vi "Promedio.vi"(0 "Datos_IN":dbl[][](array[numeric]), 5 "Error In":errorcluster) -> (14 "Prom_Array":dbl[](array[numeric]), 19 "Error Out":errorcluster)   [LabVIEW 2013]
doc: "Finds the median value of the input sequence X by sorting the values of X and averaging the middle element(s) of the sorted array."
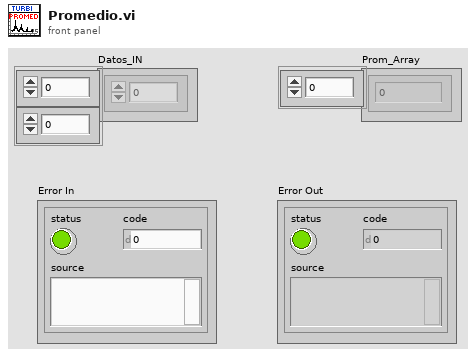
[diagram p1: front panel]
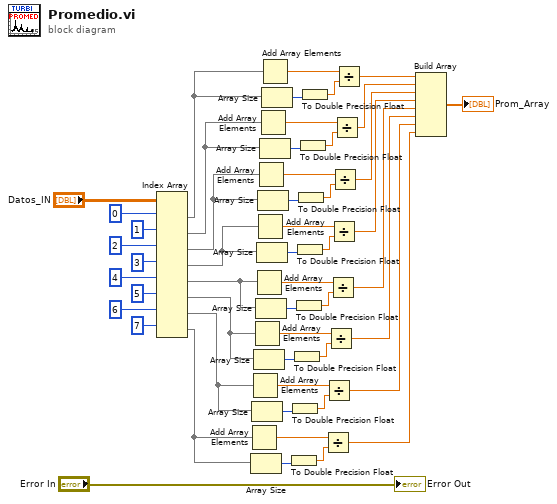
[diagram p0: block diagram]
diagram:
  n1 = Index Array(array="Datos_IN", index (row) #1=0 ("disabled index (col)"), index (row) #2=1 ("index (col)"), index (row) #3=2 ("index (col)"), index (row) #4=3 ("index (col)"), index (row) #5=4 ("index (col)"), index (row) #6=5 ("index (col)"), index (row) #7=6 ("index (col)"), index (row) #8=7 ("index (col)")) -> (element #1=w37:dbl[], element #2=w14:dbl[], element #3=w6:dbl[], element #4=w5:dbl[], element #5=w4:dbl[], element #6=w3:dbl[], element #7=w2:dbl[], element #8=w1:dbl[])  [unwired: 8 in]
  n2 = Add Array Elements(numeric array=w1) -> (sum=w17:dbl)
  n3 = Add Array Elements(numeric array=w2) -> (sum=w20:dbl)
  n4 = Array Size(array=w1) -> (size(s)=w15:i32)
  n5 = Add Array Elements(numeric array=w3) -> (sum=w23:dbl)
  n6 = Array Size(array=w2) -> (size(s)=w18:i32)
  n7 = Add Array Elements(numeric array=w4) -> (sum=w26:dbl)
  n8 = Array Size(array=w3) -> (size(s)=w21:i32)
  n9 = Add Array Elements(numeric array=w5) -> (sum=w29:dbl)
  n10 = Add Array Elements(numeric array=w6) -> (sum=w32:dbl)
  n11 = Array Size(array=w4) -> (size(s)=w24:i32)
  n12 = Array Size(array=w5) -> (size(s)=w27:i32)
  n13 = Add Array Elements(numeric array=w14) -> (sum=w35:dbl)
  n14 = Array Size(array=w6) -> (size(s)=w30:i32)
  n15 = Add Array Elements(numeric array=w37) -> (sum=w40:dbl)
  n16 = Array Size(array=w14) -> (size(s)=w33:i32)
  n17 = Array Size(array=w37) -> (size(s)=w38:i32)
  n18 = To Double Precision Float(number=w15) -> (double precision float=w16:dbl)
  n19 = To Double Precision Float(number=w18) -> (double precision float=w19:dbl)
  n20 = To Double Precision Float(number=w21) -> (double precision float=w22:dbl)
  n21 = To Double Precision Float(number=w24) -> (double precision float=w25:dbl)
  n22 = To Double Precision Float(number=w27) -> (double precision float=w28:dbl)
  n23 = To Double Precision Float(number=w30) -> (double precision float=w31:dbl)
  n24 = To Double Precision Float(number=w33) -> (double precision float=w34:dbl)
  n25 = To Double Precision Float(number=w38) -> (double precision float=w39:dbl)
  n26 = Divide(x=w17, y=w16) -> (x/y=w7:dbl)
  n27 = Divide(x=w20, y=w19) -> (x/y=w8:dbl)
  n28 = Divide(x=w23, y=w22) -> (x/y=w9:dbl)
  n29 = Divide(x=w26, y=w25) -> (x/y=w10:dbl)
  n30 = Divide(x=w29, y=w28) -> (x/y=w11:dbl)
  n31 = Divide(x=w32, y=w31) -> (x/y=w12:dbl)
  n32 = Divide(x=w35, y=w34) -> (x/y=w13:dbl)
  n33 = Divide(x=w40, y=w39) -> (x/y=w36:dbl)
  n34 = Build Array(w36, w13, w12, w11, w10, w9, w8, w7) -> (→"Prom_Array":dbl[])
  "Error Out" <- "Error In"
